vi "BP RT Save.vi"(8 "error in":errorcluster, 10 "View Model in":T1, 11 "TDMS in":refnum<class "TDMS.lvclass">) -> (0 "error out":errorcluster, 3 "TDMS out":refnum<class "TDMS.lvclass">)   [LabVIEW 2017, in "Report_lib.lvlib" / "TDMS.lvclass"]
doc: "This SubVI prepare and store the portion of DAQ data (one record) in the opened TDMS file"
uses:
  TDMS.lvclass
  View Model/Controls/View Model.ctl
  View Model/Controls/Shared Model.ctl
  Error Handler/Controls/Error Model.ctl
  Error Handler/Controls/Error Event.ctl
  Error Handler/Controls/Error Type.ctl
  Controller/Controls/Controller Model.ctl
  Controller/Controls/Controller Event.ctl
  Controller/Controls/Controller Command.ctl
  Controller/Controls/Controller Overhead.ctl
  Real-Time/RT Status.ctl
  Real-Time/RT Loop Status.ctl
  Controller/Controls/Controller NStream.ctl
  Controller/Controls/Controller Timer Data.ctl
  Controller/Controls/Controller DAQ Data.ctl
  TDMS Logger/Controls/TDMS Model.ctl
  TDMS Logger/Controls/TDMS Event.ctl
  TDMS Logger/Controls/TDMS Command.ctl
  TDMS Logger/Controls/TDMS Overhead.ctl
  TDMS Logger/Controls/TDMS ChanProperties.ctl
  TDMS Logger/Controls/TDMS DAQ Data.ctl
  TDMS.lvclass/TDMS.ctl
panel:
  out "TDMS index":i32
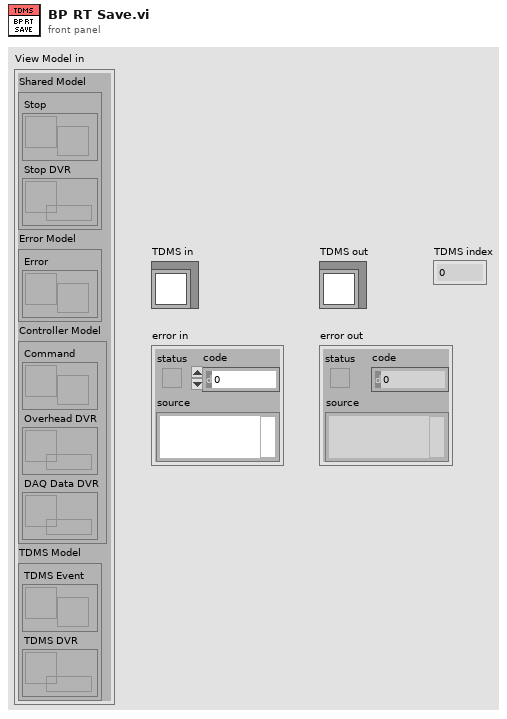
[diagram p1: front panel]
types:
  T1 = typedef "View Model.ctl" = cluster{"Shared Model":T2, "Error Model":T3, "Controller Model":T4, "TDMS Model":T5}
  T2 = typedef "Shared Model.ctl" = cluster{"Stop":refnum<user-event>, "Stop DVR":refnum<data-value>}
  T3 = typedef "Error Model.ctl" = cluster{"Error":refnum<user-event>}
  T4 = typedef "Controller Model.ctl" = cluster{"Command":refnum<user-event>, "Overhead DVR":refnum<data-value>, "DAQ Data DVR":refnum<data-value>}
  T5 = typedef "TDMS Model.ctl" = cluster{"TDMS Event":refnum<user-event>, "TDMS DVR":refnum<data-value>}
  T6 = typedef "TDMS DAQ Data.ctl" = cluster{"AOM data":dbl[], "AIMV data":dbl[], "AIMC data":dbl[], "DOM data":dbl[], "DIM data":dbl[], "AOM timestamp":dbl, "AIMV timestamp":dbl, "AIMC timestamp":dbl, "DOM timestamp":dbl, "DIM timestamp":dbl}
  T7 = typedef "TDMS ChanProperties.ctl" = cluster{"AOM9":string[][], "AIM2":string[][], "DIM3":string[][], "DIM4":string[][], "DOM6":string[][], "DOM7":string[][]}
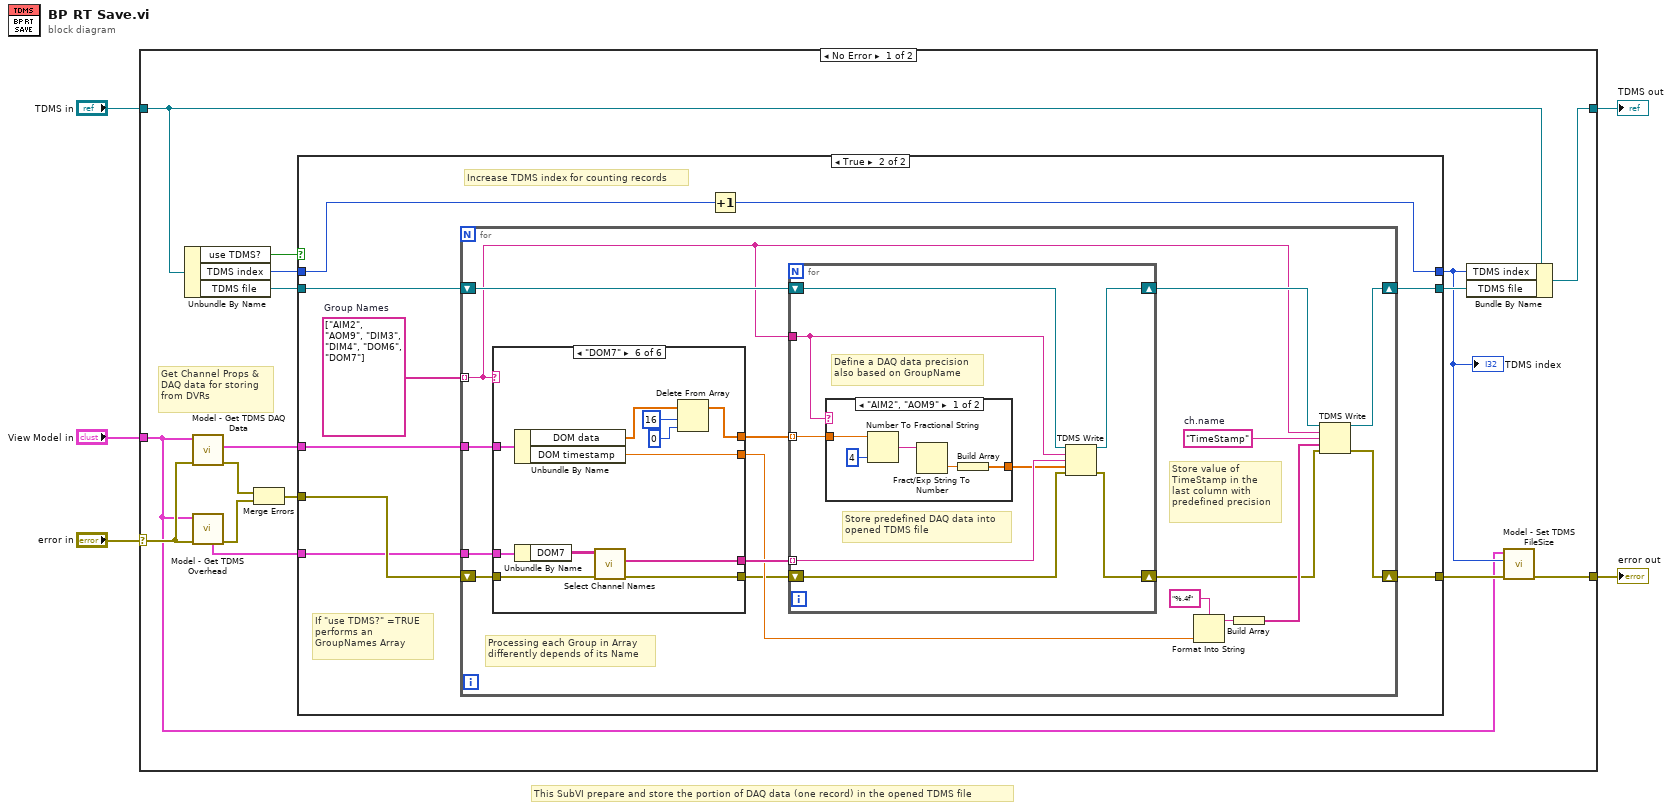
[diagram p0: block diagram]
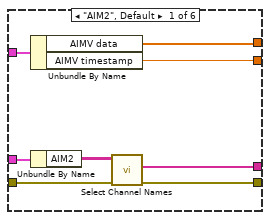
[diagram p3: hidden frame]
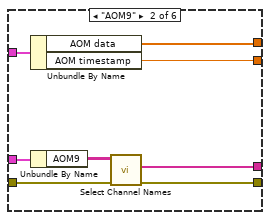
[diagram p4: hidden frame]
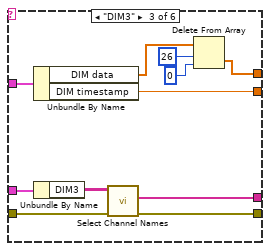
[diagram p5: hidden frame]
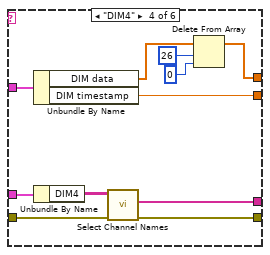
[diagram p6: hidden frame]
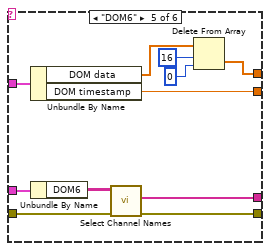
[diagram p7: hidden frame]
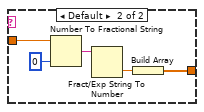
[diagram p8: hidden frame]
diagram:
  # "This SubVI prepare and store the portion of DAQ data (one record) in the opened TDMS file"
  n1 = case shown="No Error" "error in" {
    selector: "error in" -> [w15 w130]
    tunnel: [w8 w130] -> w2
    tunnel: [w17 w129] -> w3
    tunnel: "TDMS in" -> [w18 w129]
    tunnel: "View Model in" -> [w6 _]
    frame No Error {
      # "Get Channel Props &\nDAQ data for storing\nfrom DVRs"
      n2 = Unbundle By Name(w18) -> ("use TDMS?"=w10:bool, "TDMS index"=w20:i32, "TDMS file"=w21:refnum<k34>)
      n3 = call "Model - Get TDMS DAQ Data.vi"("error in (no error)"=w15, "View Model"=w6) -> ("error out"=w11:errorcluster, "TDMS DAQ Data"=w14:T6)  [unwired: 7 in, 1 out]
      n4 = call "Model - Get TDMS Overhead.vi"("error in (no error)"=w15, "View Model"=w6) -> ("error out"=w12:errorcluster, "ChProps"=w16:T7)  [unwired: 4 in, 4 out]
      n5 = Merge Errors(w11, w12) -> (w13:errorcluster)
      n6 = case shown="True" w10 {
        tunnel: w21 -> [w23 w32]
        tunnel: w13 -> [w22 w31]
        tunnel: w20 -> [w24 w30]
        tunnel: [w24 w29] -> w7
        tunnel: [w23 w28] -> w19
        tunnel: w14 -> [_ w27]
        tunnel: [w22 w26] -> w9
        tunnel: w16 -> [_ w25]
        frame False {
        }
        frame True {
          w33 = string[] ["AIM2", "AOM9", "DIM3", "DIM4", "DOM6", "DOM7"]  # Group Names
          # "Increase TDMS index for counting records"
          # "If \"use TDMS?\" =TRUE\nperforms an \nGroupNames Array"
          n7 = for {
            tunnel: w33 -> [w36] mode=indexing
            tunnel: w25 -> [w49]
            tunnel: w27 -> [w50]
            shift-right: [w38] -> w28
            shift-left: w32 -> [w46]
            shift-right: [w37] -> w26
            shift-left: w31 -> [w35]
            w45 = "TimeStamp"  # ch.name
            # "Store value of\nTimeStamp in the\nlast column with\npredefined precision"
            # "Processing each Group in Array\ndifferently depends of its Name"
            n8 = case shown="\"DOM7\"" w36 {
              tunnel: w50 -> [w58 w66 w77 w88 w99 w110]
              tunnel: w49 -> [w57 w65 w76 w87 w98 w109]
              tunnel: [w56 w64 w72 w83 w94 w104] -> w48
              tunnel: [w53 w61 w69 w80 w91 w102] -> w47
              tunnel: [w55 w63 w75 w86 w97 w108] -> w40
              tunnel: w35 -> [w52 w60 w68 w79 w90 w101]
              tunnel: [w51 w59 w67 w78 w89 w100] -> w34
              frame "AIM2", Default {
                n9 = Unbundle By Name(w58) -> ("AIMV data"=w56:dbl[], "AIMV timestamp"=w55:dbl)
                n10 = Unbundle By Name(w57) -> ("AIM2"=w54:string[][])
                n11 = call "Select Channel Names.vi"("error in (no error)"=w52, "2D Channel Params"=w54) -> ("error out"=w51:errorcluster, "Ch.Names"=w53:string[])  [unwired: 7 in, 1 out]
              }
              frame "AOM9" {
                n12 = Unbundle By Name(w66) -> ("AOM data"=w64:dbl[], "AOM timestamp"=w63:dbl)
                n13 = Unbundle By Name(w65) -> ("AOM9"=w62:string[][])
                n14 = call "Select Channel Names.vi"("error in (no error)"=w60, "2D Channel Params"=w62) -> ("error out"=w59:errorcluster, "Ch.Names"=w61:string[])  [unwired: 7 in, 1 out]
              }
              frame "DIM3" {
                n15 = Unbundle By Name(w77) -> ("DIM data"=w71:dbl[], "DIM timestamp"=w75:dbl)
                n16 = Unbundle By Name(w76) -> ("DIM3"=w70:string[][])
                n17 = call "Select Channel Names.vi"("error in (no error)"=w68, "2D Channel Params"=w70) -> ("error out"=w67:errorcluster, "Ch.Names"=w69:string[])  [unwired: 7 in, 1 out]
                n18 = Delete From Array(array=w71, length=26, index=0) -> (deleted portion=w72:dbl[])  [unwired: 1 out]
              }
              frame "DIM4" {
                n19 = Unbundle By Name(w88) -> ("DIM data"=w82:dbl[], "DIM timestamp"=w86:dbl)
                n20 = Unbundle By Name(w87) -> ("DIM4"=w81:string[][])
                n21 = call "Select Channel Names.vi"("error in (no error)"=w79, "2D Channel Params"=w81) -> ("error out"=w78:errorcluster, "Ch.Names"=w80:string[])  [unwired: 7 in, 1 out]
                n22 = Delete From Array(array=w82, length=26, index=0) -> (array with subset deleted=w83:dbl[])  [unwired: 1 out]
              }
              frame "DOM6" {
                n23 = Unbundle By Name(w99) -> ("DOM data"=w93:dbl[], "DOM timestamp"=w97:dbl)
                n24 = Unbundle By Name(w98) -> ("DOM6"=w92:string[][])
                n25 = call "Select Channel Names.vi"("error in (no error)"=w90, "2D Channel Params"=w92) -> ("error out"=w89:errorcluster, "Ch.Names"=w91:string[])  [unwired: 7 in, 1 out]
                n26 = Delete From Array(array=w93, length=16, index=0) -> (deleted portion=w94:dbl[])  [unwired: 1 out]
              }
              frame "DOM7" {
                n27 = Unbundle By Name(w110) -> ("DOM data"=w107:dbl[], "DOM timestamp"=w108:dbl)
                n28 = Unbundle By Name(w109) -> ("DOM7"=w103:string[][])
                n29 = call "Select Channel Names.vi"("error in (no error)"=w101, "2D Channel Params"=w103) -> ("error out"=w100:errorcluster, "Ch.Names"=w102:string[])  [unwired: 7 in, 1 out]
                n30 = Delete From Array(array=w107, length=16, index=0) -> (array with subset deleted=w104:dbl[])  [unwired: 1 out]
              }
            }
            n31 = for {
              tunnel: w48 -> [w118] mode=indexing
              tunnel: w47 -> [w115] mode=indexing
              shift-right: [w116] -> w42
              shift-left: w46 -> [w117]
              tunnel: w36 -> [w111]
              shift-right: [w112] -> w43
              shift-left: w34 -> [w113]
              # "Store predefined DAQ data into\nopened TDMS file"
              # "Define a DAQ data precision\nalso based on GroupName"
              n32 = case shown="\"AIM2\", \"AOM9\"" w111 {
                tunnel: w118 -> [w120 w125]
                tunnel: [w119 w124] -> w114
                frame "AIM2", "AOM9" {
                  n33 = Number To Fractional String(number=w120, precision (6)=i16 4) -> (F-format string=w122:string)  [unwired: 2 in]
                  n34 = Fract/Exp String To Number(string=w122) -> (number=w123:dbl)  [unwired: 3 in, 1 out]
                  n35 = Build Array(w123) -> (w119:dbl[])
                }
                frame Default {
                  n36 = Number To Fractional String(number=w125, precision (6)=i16 0) -> (F-format string=w127:string)  [unwired: 2 in]
                  n37 = Fract/Exp String To Number(string=w127) -> (number=w128:dbl)  [unwired: 3 in, 1 out]
                  n38 = Build Array(w128) -> (w124:dbl[])
                }
              }
              n39 = TDMS Write(0:w117, 5:w111, 7:w115, 9:w114, 11:w113) -> (4:w116:refnum<k34>, 15:w112:errorcluster)  [unwired: 1 in, 2 out]
            }
            n40 = Format Into String(format string="%.4f", w40) -> (resulting string=w39:string)  [unwired: 2 in, 1 out]
            n41 = Build Array(w39) -> (w44:string[])
            n42 = TDMS Write(0:w42, 5:w36, 7:w45, 9:w44, 11:w43) -> (4:w38:refnum<k34>, 15:w37:errorcluster)  [unwired: 1 in, 2 out]
          }
          n43 = Increment(x=w30) -> (x+1=w29:i32)
        }
      }
      "TDMS index" <- w7
      n44 = Bundle By Name(cluster=w18, "TDMS index"=w7, "TDMS file"=w19) -> (w17:refnum<class "TDMS.lvclass">)
      n45 = call "Model - Set TDMS FileSize.vi"("error in (no error)"=w9, "FileSize"=w7, "View Model"=w6) -> ("error out"=w8:errorcluster)  [unwired: 7 in, 1 out]
    }
    frame Error {
    }
  }
  "error out" <- w2
  "TDMS out" <- w3
